vi "uninstall tag bus.vi"   [LabVIEW 2013]
uses:
  <vilib>/JKI/VIPM API/VIPM API_vipm_api.lvlib
types:
  T1 = typedef "VIPM API_vipm_api.lvlib/VI Package Build Spec Data Cluster_vipm_api.ctl" = cluster{"Package Version":T2, "Product Name":string, "Company Name":string, "Author Name (Person or Company)":string, "Product Homepage (URL)":string, "Legal Copyright":string, "License Agreement Name":string, "Product Description Summary":string, "Product Description":string, "Release Notes - Change Log":string}
  T2 = typedef "VIPM API_vipm_api.lvlib/Version Info Cluster_vipm_api.ctl" = cluster{"major":u32, "minor":u32, "patch":u32, "build":u32}
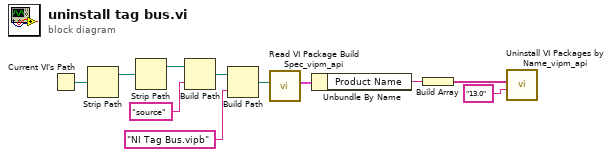
[diagram p0: block diagram]
diagram:
  n1 = Current VI's Path() -> (path=w7:path)
  n2 = Strip Path(path=w7) -> (stripped path=w6:path)  [unwired: 1 out]
  n3 = Strip Path(path=w6) -> (stripped path=w4:path)  [unwired: 1 out]
  n4 = Build Path(base path=w4, name or relative path="source") -> (appended path=w2:path)
  n5 = Build Path(base path=w2, name or relative path="NI Tag Bus.vipb") -> (appended path=w1:path)
  n6 = call <vilib>:"Read VI Package Build Spec_vipm_api.vi"("Path to VIPB File"=w1) -> ("VI Package Build Spec Data"=w10:T1)  [unwired: 9 in, 1 out]
  n7 = Unbundle By Name(w10) -> ("Product Name"=w9:string)
  n8 = Build Array(w9) -> (w8:string[])
  n9 = call <vilib>:"Uninstall VI Packages by Name_vipm_api.vi"("LabVIEW Version"="13.0", "Package Names to Uninstall []"=w8) -> ()  [unwired: 9 in, 1 out]
